vi "文本文件（格式化读取）.vi"() -> ()   [LabVIEW 2017]
panel:
  out "波形图":dbl[](graph)
  out "数组":timestamp[](array[timestamp])
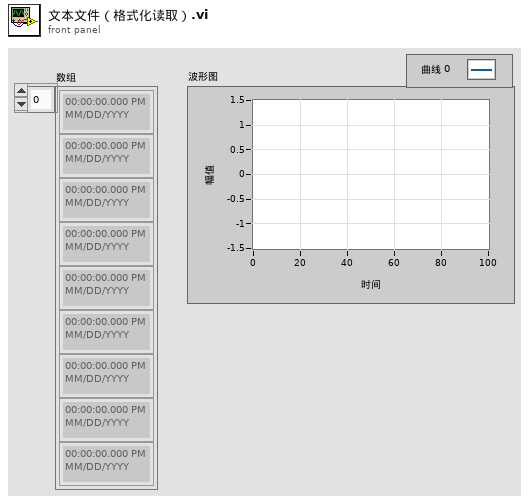
[diagram p1: front panel]
types:
  T1 = enum16{"open", "replace", "create", "open or create", "replace or create", "replace or create with confirmation"}
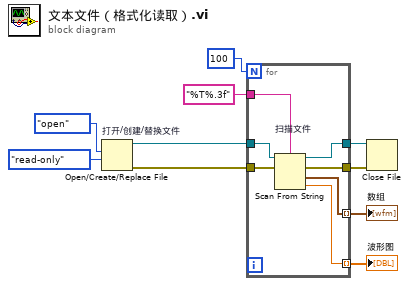
[diagram p0: block diagram]
diagram:
  n1 = Open/Create/Replace File "打开/创建/替换文件"(operation (0:open)=T1."open" ("操作(0:open)"), access (0:read/write)=enum16{"read/write", "read-only", "write-only"}."read-only" ("权限(0:read/write)")) -> (refnum out=w9:refnum<file>, error out=w8:errorcluster)  [unwired: 4 in, 1 out]
  n2 = for {
    N: 100 -> [_]
    tunnel: w9 -> [w17]
    tunnel: w8 -> [w16]
    tunnel: "%T%.3f" ("格式字符串") -> [w15]
    tunnel: [w14] -> w6
    tunnel: [w13] -> w5
    tunnel: [w12] -> w4 mode=indexing
    tunnel: [w11] -> w3 mode=indexing
    n3 = Scan From String "扫描文件"(w15, w17, w16) -> (w14:refnum<file>, w13:errorcluster, output 1=w12:timestamp, output 2=w11:dbl)  [unwired: 2 in]
  }
  "数组" <- w4
  "波形图" <- w3
  n4 = Close File(refnum=w6, error in=w5) -> ()  [unwired: 2 out]
